vi "HDF5_Write_Noise_Trace.vi"(0 "NoiseRef":T1 {"TimeStamp_df_dset" format="%.0x"; "sum_dset" format="%.0x"; "df_dset" format="%.0x"; "TimeStamp_dset" format="%.0x"; "SumdSpectrum_dset" format="%.0x"; "TimeString_dset" format="%.0x"; "Group_ref" format="%.0x"}, 7 "NoiseTrace":dbl[](array[numeric]), 11 "error in":errorcluster) -> (15 "error out":errorcluster)   [LabVIEW 2018]
doc: "Write a single Noise<x> record with timestamp:\nNoise1\n NoiseInfo - cluster with Timestamp and other metadata for this record\n SummdSpectrum - 1024 element Double array (waveform)"
uses:
  HDF5_Noise_refs.ctl
  <vilib>/addons/h5labview2/base/hid_t.ctl
  lib_path_mod_20200519.vi
  <vilib>/addons/h5labview2/base/H5Equery.vi
  <vilib>/addons/h5labview2/dataset/H5Dwrite.llb/H5Dwrite.xnode
  <vilib>/addons/h5labview2/dataset/H5D.lvlib
  <vilib>/addons/h5labview2/space/H5S.lvlib
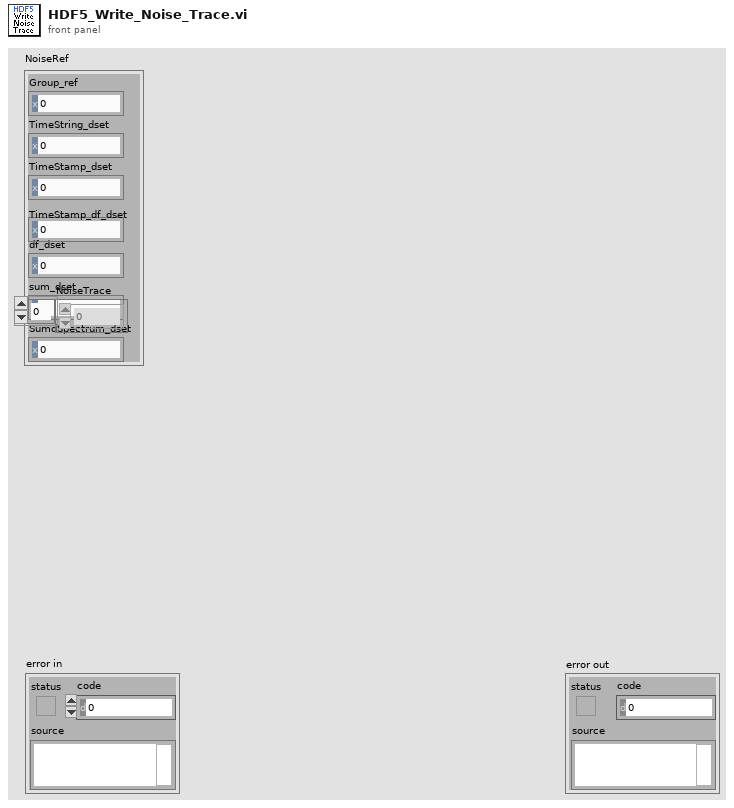
[diagram p1: front panel]
types:
  T1 = typedef "HDF5_Noise_refs.ctl" = cluster{"Group_ref":T2, "TimeString_dset":T2, "TimeStamp_dset":T2, "TimeStamp_df_dset":T2, "df_dset":T2, "sum_dset":T2, "SumdSpectrum_dset":T2}
  T2 = typedef "hid_t.ctl" = i32
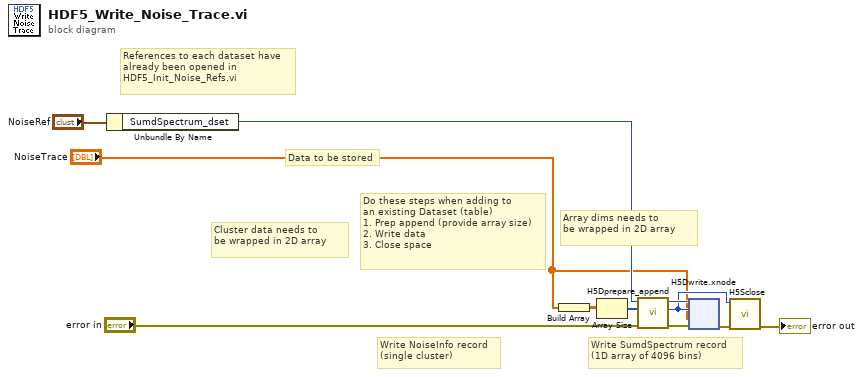
[diagram p0: block diagram]
diagram:
  # "Array dims needs to \nbe wrapped in 2D array"
  # "Cluster data needs to \nbe wrapped in 2D array"
  # "Data to be stored"
  # "References to each dataset have \nalready been opened in \nHDF5_Init_Noise_Refs.vi"
  # "Do these steps when adding to \nan existing Dataset (table)\n1. Prep append (provide array size)\n2. Write data\n3. Close space"
  # "Write SumdSpectrum record\n(1D array of 4096 bins)"
  # "Write NoiseInfo record\n(single cluster)"
  n1 = Unbundle By Name("NoiseRef") -> ("SumdSpectrum_dset"=w5:T2)
  n2 = Build Array("NoiseTrace") -> (w2:dbl[][])
  n3 = Array Size(array=w2) -> (size(s)=w4:i32[])
  n4 = call <vilib>:"H5Dprepare_append.vi"("error in (no error)"="error in", "append dims"=w4, "dset in"=w5) -> ("error out"=w9:errorcluster, "space out"=w10:T2, "dset out"=w11:T2)  [unwired: 5 in, 1 out]
  n5 = xnode "H5Dwrite.xnode"("error in (no error)"=w9, "data"="NoiseTrace", "file space"=w10, "ref in"=w11) -> ("error out"=w8:errorcluster)  [unwired: 3 in, 2 out]
  n6 = call <vilib>:"H5Sclose.vi"("error in (no error)"=w8, "space in"=w10) -> ("error out"=→"error out":errorcluster)  [unwired: 9 in]
